vi "Get Position For Align Or Distribute.vi"(8 "Error In":errorcluster, 10 "Vertical? (F: Horizontal)":bool, 11 "Splitter in":refnum<class "Splitter.lvclass">) -> (0 "Error Out":errorcluster, 1 "Position":i32, 2 "Applicable?":bool, 3 "Splitter out":refnum<class "Splitter.lvclass">)   [LabVIEW 2017, in "Splitter.lvclass"]
uses:
  Splitter.lvclass
  Splitter.lvclass/Splitter.ctl
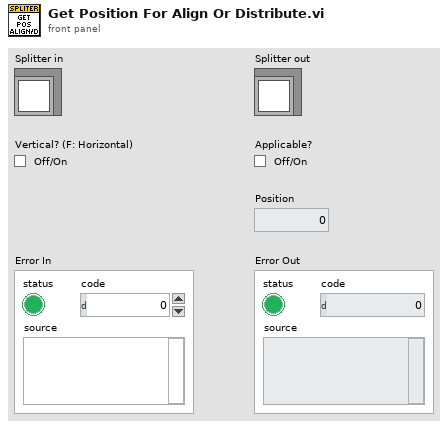
[diagram p1: front panel]
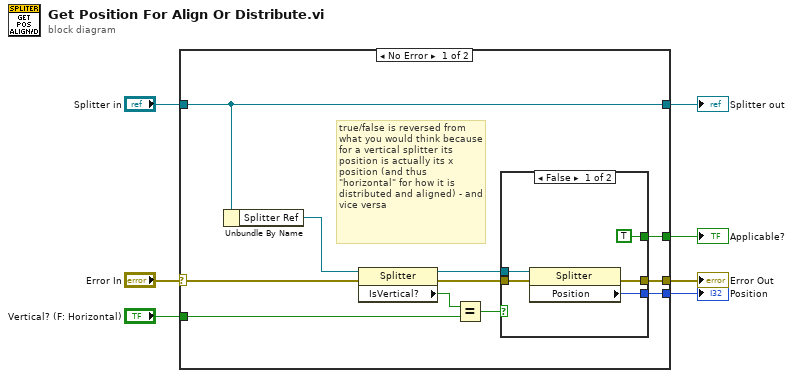
[diagram p0: block diagram]
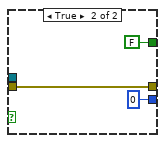
[diagram p2: hidden frame]
diagram:
  n1 = case shown="No Error" "Error In" {
    selector: "Error In" -> [w17 w27]
    tunnel: "Splitter in" -> [w14 w28]
    tunnel: [w9 w27] -> w5
    tunnel: "Vertical? (F: Horizontal)" -> [w15 _]
    tunnel: [w14 w28] -> w3
    tunnel: [w10 _] -> w2
    tunnel: [w8 _] -> w1
    frame No Error {
      # "true/false is reversed from what you would think because for a vertical splitter its position is actually its x position (and thus \"horizontal\" for how it is distributed and aligned) - and vice versa"
      n2 = Unbundle By Name(w14) -> ("Splitter Ref"=w18:refnum<vi>)
      n3 = property class="Splitter"(reference=w18, error in=w17) -> (reference out=w11:refnum<vi>, error out=w13:errorcluster, "IsVertical?"=w16:bool)
      n4 = Equal?(x=w16, y=w15) -> (x = y?=w12:bool)
      n5 = case shown="False" w12 {
        tunnel: w13 -> [w23 w25]
        tunnel: w11 -> [w22 _]
        tunnel: [w21 0 ("Position")] -> w10
        tunnel: [w20 w25] -> w9
        tunnel: [TRUE FALSE] -> w8
        frame False {
          n6 = property class="Splitter"(reference=w22, error in=w23) -> (error out=w20:errorcluster, "Position"=w21:i32)  [unwired: 1 out]
        }
        frame True {
        }
      }
    }
    frame Error {
    }
  }
  "Splitter out" <- w3
  "Error Out" <- w5
  "Applicable?" <- w1
  "Position" <- w2
